vi "set parameters.vi"(8 "error in (no error)":errorcluster, 10 "parameters":T1, 11 "Task.lvclass in":refnum<class "Task.lvclass">) -> (0 "error out":errorcluster, 3 "Task.lvclass out":refnum<class "Task.lvclass">)   [LabVIEW 2020, in "Tasks.lvlib" / "Task.lvclass"]
uses:
  Task.lvclass
  parameters.ctl
  Task.lvclass/Task.ctl
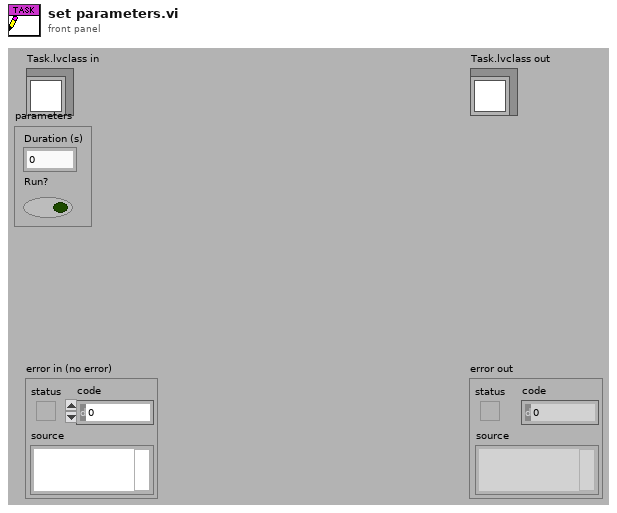
[diagram p1: front panel]
types:
  T1 = typedef "Tasks.lvlib/Task.lvclass/parameters.ctl" = cluster{"Duration (s)":dbl, "Run?":bool}
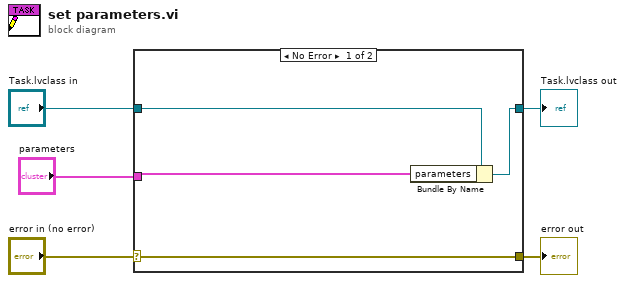
[diagram p0: block diagram]
diagram:
  n1 = case shown="No Error" "error in (no error)" {
    selector: "error in (no error)" -> [w9 w10]
    tunnel: [w9 w10] -> w4
    tunnel: [w7 w11] -> w2
    tunnel: "Task.lvclass in" -> [w8 w11]
    tunnel: "parameters" -> [w6 _]
    frame No Error {
      n2 = Bundle By Name(cluster=w8, "parameters"=w6) -> (w7:refnum<class "Task.lvclass">)
    }
    frame Error {
    }
  }
  "error out" <- w4
  "Task.lvclass out" <- w2
